vi "Update Display.vi"(8 "error in (no error)":errorcluster, 9 "Active Pixels":cluster{"Column":u8, "Row":u8, "Color":u32}[](array[cluster]), 10 "Board State":u32[][](array[numeric]), 11 "Screen Interface in":refnum<class "Screen Interface.lvclass">) -> (0 "error out":errorcluster, 3 "Screen Interface out":refnum<class "Screen Interface.lvclass">)   [LabVIEW 2017, in "Screen Interface.lvlib" / "Screen Interface.lvclass"]
uses:
  Screen Interface.lvclass
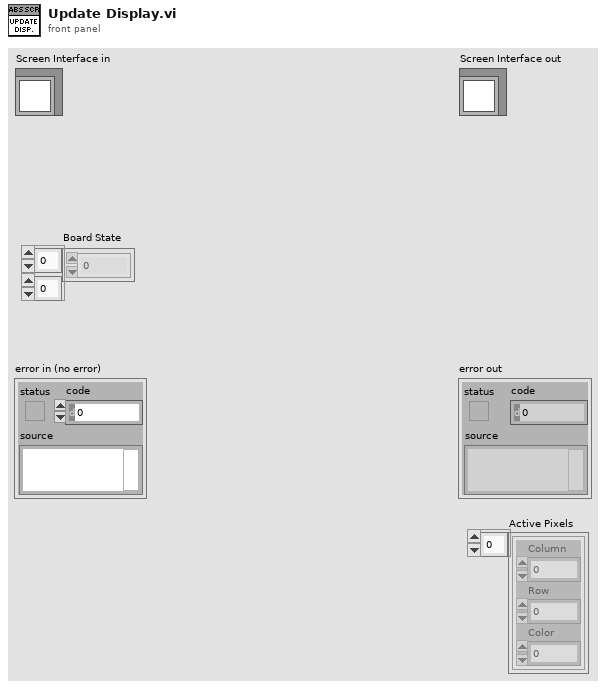
[diagram p1: front panel]
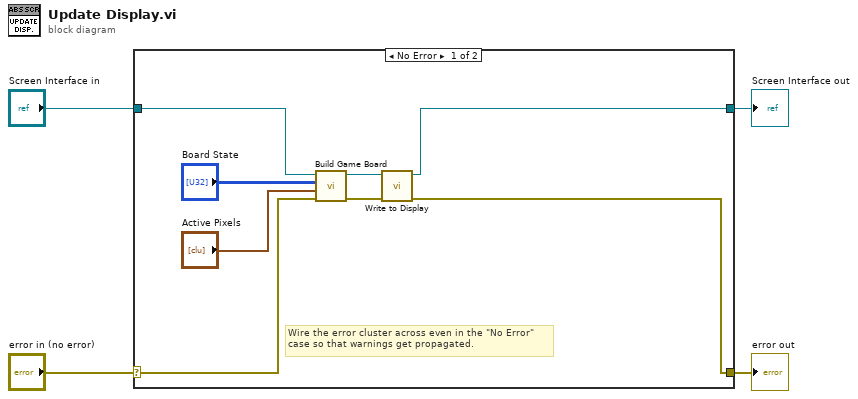
[diagram p0: block diagram]
diagram:
  n1 = case shown="No Error" "error in (no error)" {
    selector: "error in (no error)" -> [w10 w14]
    tunnel: [w5 w14] -> w3
    tunnel: [w7 w13] -> w1
    tunnel: "Screen Interface in" -> [w9 w13]
    frame No Error {
      # "Wire the error cluster across even in the \"No Error\"\ncase so that warnings get propagated."
      n2 = call-dynamic "Build Game Board.vi"("error in (no error)"=w10, "Active Pixels"="Active Pixels", "Board To Draw"="Board State", "Screen Interface in"=w9) -> ("error out"=w6:errorcluster, "Screen Interface out"=w8:refnum<class "Screen Interface.lvclass">)  [unwired: 6 in]
      n3 = call-dynamic "Write to Display.vi"("error in (no error)"=w6, "Screen Interface in"=w8) -> ("error out"=w5:errorcluster, "Screen Interface out"=w7:refnum<class "Screen Interface.lvclass">)  [unwired: 8 in]
    }
    frame Error {
    }
  }
  "error out" <- w3
  "Screen Interface out" <- w1
